vi "WSVCAP SHL FPGA LL Procedure I2C - Send ACK.vi"(0 "Procedure Step":T1, 1 "Wait Ticks Remaining":u32, 5 "I2C Wait Ticks":u32, 7 "ACK Bit to Write":bool, 11 "error in (no error)":errorcluster, 13 "Socket Mask":u64 format="%012x") -> (3 "Wait Ticks Remaining Out":u32, 4 "Procedure Step Out":T1, 8 "Finished":bool, 15 "error out":errorcluster)   [LabVIEW 2012]
uses:
  Type Defs/WSVCAP SHL Procedure Step Enum.ctl
  Type Defs/WSVCAP SHL I2C Write Line Enum.ctl
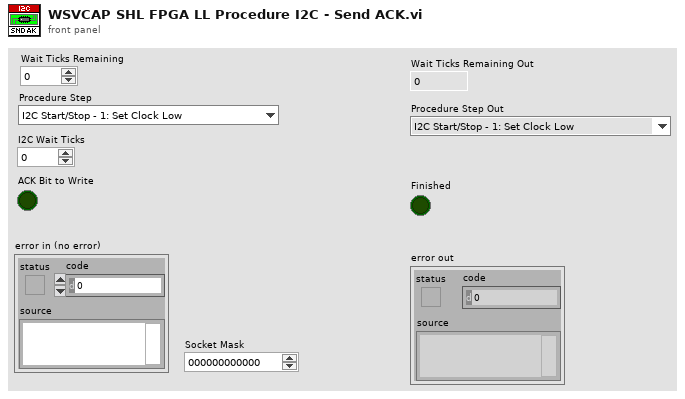
[diagram p1: front panel]
types:
  T1 = typedef "WSVCAP SHL Procedure Step Enum.ctl" = enum16{"I2C Start/Stop - 1: Set Clock Low", "I2C Start/Stop - 2: Wait", "I2C Start/Stop - 3: Set Data I", "I2C Start/Stop - 4: Wait", "I2C Start/Stop - 5: Set Clock High", "I2C Start/Stop - 6: Wait", "I2C Start/Stop - 7: Set Data II", "I2C Start/Stop - 8: Wait", "I2C Start/Stop - 9: Set Clock Low", "I2C Start/Stop - 10: Wait", "I2C Read ACK - 1: Set Clock High", "I2C Read ACK - 2: Wait", "I2C Read ACK - 3: Read ACK Bit", "I2C Read ACK - 4: Wait", "I2C Read ACK - 5: Set Clock Low", "I2C Read ACK - 6: Wait", "I2C Write ACK - 1: Write ACK Bit", "I2C Write ACK - 2: Wait", "I2C Write ACK - 3: Set Clock High", "I2C Write ACK - 4: Wait", "I2C Write ACK - 5: Set Clock Low", "I2C Write ACK - 6: Wait", "I2C Write ACK - 7: Set Data Low", "I2C Send Add - 1: Reset Bits Remaining", "I2C Send Add - 2: Set Data Bit", "I2C Send Add - 3: Wait", "I2C Send Add - 4: Set Clock High", "I2C Send Add - 5: Wait", "I2C Send Add - 6: Set Clock Low", "I2C Send Add - 7: Wait", "I2C Send Add - 8: Check Bits Remaining", "I2C Send Data - 1: Reset Bits Remaining", "I2C Send Data - 2: Load Write Bit from FIFO", "I2C Send Data - 3: Set Data Bit", "I2C Send Data - 4: Wait", "I2C Send Data - 5: Set Clock High", "I2C Send Data - 6: Wait", "I2C Send Data - 7: Set Clock Low", "I2C Send Data - 8: Wait", "I2C Send Data - 9: Check Bits Remaining", "I2C Receive Data - 1: Reset Bits Remaining", "I2C Receive Data - 2: Wait", "I2C Receive Data - 3: Set Clock High", "I2C Receive Data - 4: Wait", "I2C Receive Data - 5: Read Data Bit", "I2C Receive Data - 6: Wait", "I2C Receive Data - 7: Set Clock Low", "I2C Receive Data - 8: Wait", "I2C Receive Data - 9: Check Bits Remaining", "SPI Clear Lines - 1:Clear", "SPI Send/Receive - 1: Load SDA - Clock Low", "SPI Send/Receive - 2: Wait", "SPI Send/Receive - 3: Load DATO - Clock High", "SPI Send/Receive - 4: Wait", "SPI Wait CMD Delay - 1:Wait", "RFFE Send SSC - 1:Set Low", "RFFE Send SSC - 2:Wait", "RFFE Send SSC - 3:Set SDA High", "RFFE Send SSC - 4:Wait", "RFFE Send SSC - 5:Set SDA Low", "RFFE Send SSC - 6:Wait", "RFFE Send Data - 1:Set SCL High", "RFFE Send Data - 2:Wait", "RFFE Send Data - 3:Set SCL Low", "RFFE Send Data - 4:Wait", "RFFE Send Data - 5:Set SCL High (P)", "RFFE Send Data - 6:Wait", "RFFE Send Data - 7:Set SCL Low (P)", "RFFE Send Data - 8:Wait", "RFFE Send Data - 9:Set SCL High (BP)", "RFFE Send Data - 10:Wait", "RFFE Send Data - 11:Set SCL Low (BP)", "RFFE Send Data - 12:Wait", "RFFE Receive Data - 1:Set SCL High", "RFFE Receive Data - 2:Wait", "RFFE Receive Data - 3:Set SCL Low", "RFFE Receive Data - 4:Wait", "RFFE Receive Data - 5:Set SCL High (BP)", "RFFE Receive Data - 6:Wait", "RFFE Receive Data - 7:Set SCL Low (BP)", "RFFE Receive Data - 8:Wait", "RFFE Wait CMD Delay - 1:Wait", "RFFE Clear Lines - 1:Clear"}
  T2 = typedef "WSVCAP SHL I2C Write Line Enum.ctl" = enum16{"I2C SCL", "I2C SDA"}
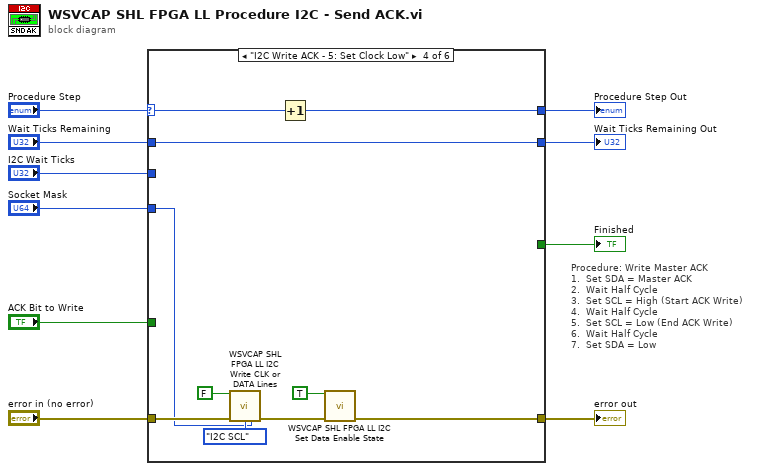
[diagram p0: block diagram]
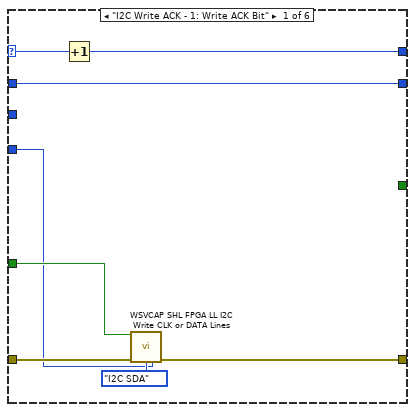
[diagram p2: hidden frame]
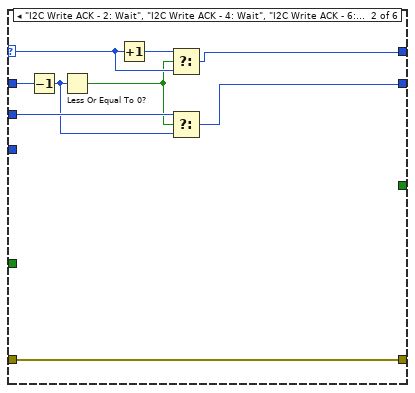
[diagram p3: hidden frame]
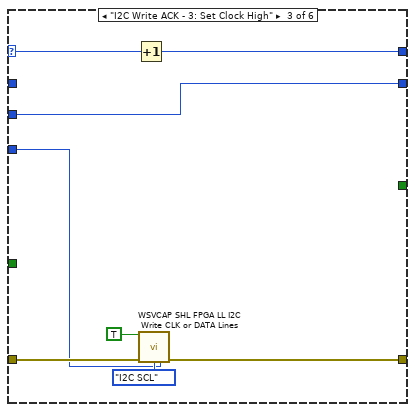
[diagram p4: hidden frame]
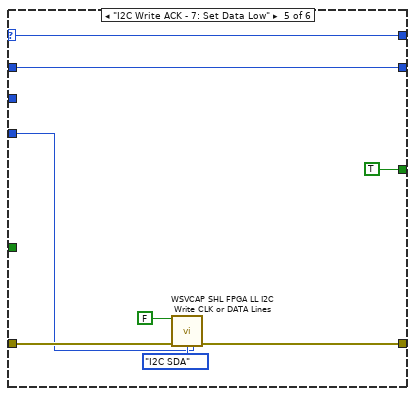
[diagram p5: hidden frame]
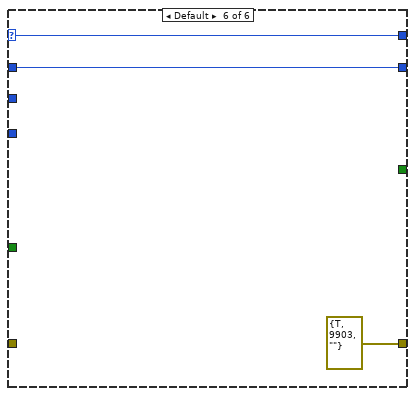
[diagram p6: hidden frame]
diagram:
  # "Procedure: Write Master ACK\n1.  Set SDA = Master ACK\n2.  Wait Half Cycle\n3.  Set SCL = High (Start ACK Write)\n4.  Wait Half Cycle\n5.  Set SCL = Low (End ACK Write)\n6.  Wait Half Cycle\n7.  Set SDA = Low"
  n1 = case shown="\"I2C Write ACK - 5: Set Clock Low\"" "Procedure Step" {
    selector: "Procedure Step" -> [w16 w22 w32 w39 w47 w55]
    tunnel: [w17 w25 w31 w41 w50 errorcluster {"status"=TRUE, "code"=9903, "source"=""} ("error out")] -> w9
    tunnel: "error in (no error)" -> [w18 w25 w34 w44 w51 _]
    tunnel: "Wait Ticks Remaining" -> [w11 w27 _ w36 w46 w54]
    tunnel: "I2C Wait Ticks" -> [_ w24 w28 _ _ _]
    tunnel: [_ _ _ _ TRUE _] -> w8
    tunnel: "ACK Bit to Write" -> [w15 _ _ _ _ _]
    tunnel: "Socket Mask" -> [w13 _ w30 w38 w48 _]
    tunnel: [w12 w20 w29 w37 w47 w55] -> w2
    tunnel: [w11 w19 w28 w36 w46 w54] -> w1
    frame "I2C Write ACK - 1: Write ACK Bit" {
      n2 = Increment(x=w16) -> (x+1=w12:T1)
      n3 = call "WSVCAP SHL FPGA LL I2C Write CLK or DATA Lines.vi"("Bit In"=w15, "error in (no error)"=w18, "Line"=WSVCAP_SHL_I2C_Write_Line_Enum."I2C SDA", "Socket Mask"=w13) -> ("error out"=w17:errorcluster)  [unwired: 11 in]
    }
    frame "I2C Write ACK - 2: Wait", "I2C Write ACK - 4: Wait", "I2C Write ACK - 6: Wait" {
      n4 = Decrement(x=w27) -> (x-1=w23:u32)
      n5 = Less Or Equal To 0?(x=w23) -> (x <= 0?=w21:bool)
      n6 = Increment(x=w22) -> (x+1=w26:T1)
      n7 = Select(t=w26, s=w21, f=w22) -> (s? t:f=w20:T1)
      n8 = Select(t=w24, s=w21, f=w23) -> (s? t:f=w19:u32)
    }
    frame "I2C Write ACK - 3: Set Clock High" {
      n9 = Increment(x=w32) -> (x+1=w29:T1)
      n10 = call "WSVCAP SHL FPGA LL I2C Write CLK or DATA Lines.vi"("Bit In"=TRUE, "error in (no error)"=w34, "Line"=WSVCAP_SHL_I2C_Write_Line_Enum."I2C SCL", "Socket Mask"=w30) -> ("error out"=w31:errorcluster)  [unwired: 11 in]
    }
    frame "I2C Write ACK - 5: Set Clock Low" {
      n11 = call "WSVCAP SHL FPGA LL I2C Write CLK or DATA Lines.vi"("Bit In"=FALSE, "error in (no error)"=w44, "Line"=WSVCAP_SHL_I2C_Write_Line_Enum."I2C SCL", "Socket Mask"=w38) -> ("error out"=w42:errorcluster)  [unwired: 11 in]
      n12 = Increment(x=w39) -> (x+1=w37:T1)
      n13 = call "WSVCAP SHL FPGA LL I2C Set Data Enable State.vi"("State"=TRUE, "error in (no error)"=w42) -> ("error out"=w41:errorcluster)  [unwired: 13 in]
    }
    frame "I2C Write ACK - 7: Set Data Low" {
      n14 = call "WSVCAP SHL FPGA LL I2C Write CLK or DATA Lines.vi"("Bit In"=FALSE, "error in (no error)"=w51, "Line"=WSVCAP_SHL_I2C_Write_Line_Enum."I2C SDA", "Socket Mask"=w48) -> ("error out"=w50:errorcluster)  [unwired: 11 in]
    }
    frame Default {
    }
  }
  "error out" <- w9
  "Finished" <- w8
  "Procedure Step Out" <- w2
  "Wait Ticks Remaining Out" <- w1
